vi "WaitOnHatchThenOpen.vi"   [LabVIEW 2018]
uses:
  Framework/Robot Global Data.vi
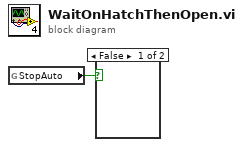
[diagram p0: block diagram]
diagram:
  n1 = global read "Robot Global Data.vi" "StopAuto"() -> (w1:bool)
  n2 = case shown="False" w1 {
    frame False {
    }
    frame True {
    }
  }
